vi "PIDINIT.vi"(11 "setpoint":dbl format="%.2f") -> ()   [LabVIEW 2013]
uses:
  <vilib>/addons/control/pid/pid.llb/PID (DBL).vi
  <vilib>/addons/control/pid/NI_PID_pid.lvlib
panel:
  in  "y 2":dbl=0.59
  in  "PID Gains for distance":T1={"proportional gain (Kc)"=1.0, "integral time (Ti, min)"=0.01, "derivative time (Td, min)"=0.0} {"derivative time (Td, min)" format="%.3f"; "integral time (Ti, min)" format="%.3f"; "proportional gain (Kc)" format="%.3f"}
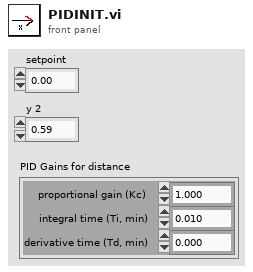
[diagram p1: front panel]
types:
  T1 = cluster{"proportional gain (Kc)":dbl, "integral time (Ti, min)":dbl, "derivative time (Td, min)":dbl}
  T2 = typedef "WPI_EncoderDevRef.ctl" = cluster{"DevStatus":errorcluster, "EncoderIndex":T3, "CounterIndex":T4, "DistancePerCount":dbl, "Decoding Type":T5}
  T3 = typedef "FPGA_EncoderIdx.ctl" = enum8{"Enc 0", "Enc 1", "Enc 2", "Enc 3", "Invalid"}
  T4 = typedef "FPGA_CounterCtrSystemIndex.ctl" = enum8{"Ctr 0", "Ctr 1", "Ctr 2", "Ctr 3", "Ctr 4", "Ctr 5", "Ctr 6", "Ctr 7", "Invalid"}
  T5 = typedef "WPI_EncoderType.ctl" = enum16{"1x", "2x", "4x"}
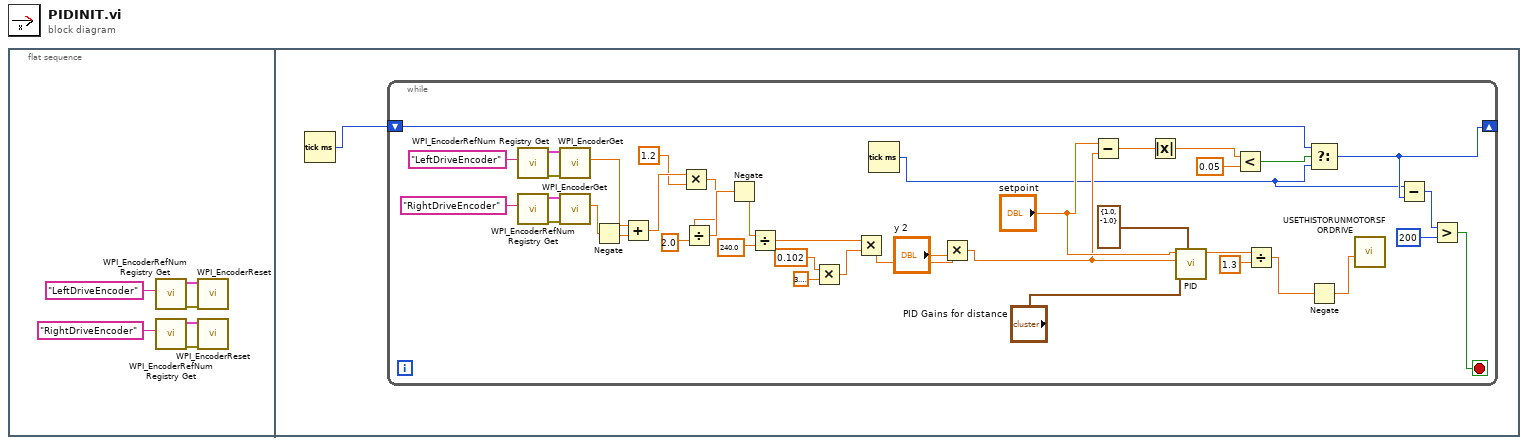
[diagram p0: block diagram]
diagram:
  n1 = flat-sequence {
    frame #0 {
      n2 = call <vilib>:"WPI_EncoderRefNum Registry Get.vi"("refnum name"="LeftDriveEncoder") -> ("error out"=w3:errorcluster, "EncoderDevRef"=w4:T2)  [unwired: 9 in]
      n3 = call <vilib>:"WPI_EncoderRefNum Registry Get.vi"("refnum name"="RightDriveEncoder") -> ("error out"=w5:errorcluster, "EncoderDevRef"=w6:T2)  [unwired: 9 in]
      n4 = call <vilib>:"WPI_EncoderReset.vi"("error in (no error)"=w3, "EncoderDevRef"=w4) -> ()  [unwired: 8 in, 2 out]
      n5 = call <vilib>:"WPI_EncoderReset.vi"("error in (no error)"=w5, "EncoderDevRef"=w6) -> ()  [unwired: 8 in, 2 out]
    }
    frame #1 {
      n6 = Tick Count (ms)() -> (millisecond timer value=w7:u32)
      n7 = while {
        shift-right: [w21] -> _
        shift-left: w7 -> [w22]
        stop <- w17 stop-if-true
        n8 = call <vilib>:"WPI_EncoderRefNum Registry Get.vi"("refnum name"="LeftDriveEncoder") -> ("error out"=w47:errorcluster, "EncoderDevRef"=w46:T2)  [unwired: 9 in]
        n9 = call <vilib>:"WPI_EncoderRefNum Registry Get.vi"("refnum name"="RightDriveEncoder") -> ("error out"=w45:errorcluster, "EncoderDevRef"=w44:T2)  [unwired: 9 in]
        n10 = call <vilib>:"WPI_EncoderGet.vi"("error in (no error)"=w47, "EncoderDevRef"=w46) -> ("Distance"=w41:dbl)  [unwired: 4 in, 5 out]
        n11 = call <vilib>:"WPI_EncoderGet.vi"("error in (no error)"=w45, "EncoderDevRef"=w44) -> ("Distance"=w14:dbl)  [unwired: 4 in, 5 out]
        n12 = Negate(x=w14) -> (-x=w13:dbl)
        n13 = Add(x=w41, y=w13) -> (x+y=w10:dbl)
        n14 = Multiply(x=w10, y=1.2) -> (x*y=w8:dbl)
        n15 = Divide(x=w8, y=2.0) -> (x/y=w12:dbl)
        n16 = Negate(x=w12) -> (-x=w11:dbl)
        n17 = Divide(x=w11, y=240.0) -> (x/y=w34:dbl)
        n18 = Multiply(x=0.102, y=3.141592653589793) -> (x*y=w36:dbl)
        n19 = Multiply(x=w34, y=w36) -> (x*y=w31:dbl)
        n20 = Tick Count (ms)() -> (millisecond timer value=w20:u32)
        n21 = Multiply(x=w31, y="y 2") -> (x*y=w27:dbl)
        n22 = Subtract(x="setpoint", y=w27) -> (x-y=w26:dbl)
        n23 = Absolute Value(x=w26) -> (abs(x)=w25:dbl)
        n24 = call-poly <vilib>:"PID.vi"("output range"=cluster{"output high":dbl, "output low":dbl} {"output high"=1.0, "output low"=-1.0}, "PID gains"="PID Gains for distance", "process variable"=w27, "setpoint"="setpoint") -> ("output"=w35:dbl)  [unwired: 6 in, 1 out]
        n25 = Less?(x=w25, y=0.05) -> (x < y?=w23:bool)
        n26 = Divide(x=w35, y=1.3) -> (x/y=w16:dbl)
        n27 = Select(t=w22, s=w23, f=w20) -> (s? t:f=w21:u32)
        n28 = Negate(x=w16) -> (-x=w15:dbl)
        n29 = call "USETHISTORUNMOTORSFORDRIVE.vi"("Y axis value"=w15) -> ()  [unwired: 11 in]
        n30 = Subtract(x=w20, y=w21) -> (x-y=w19:u32)
        n31 = Greater?(x=w19, y=u32 200) -> (0:w17:bool)
      }
    }
  }
